vi "Omron Serial FINS-Command Frame.vi"(8 "error in":errorcluster, 10 "FINS Command Frame":T3 {"Response Wait Time" items=["0 ms", "10 ms", "20 ms", "30 ms", "40 ms", "50 ms", "60 ms", "70 ms", "80 ms", "90 ms", "100 ms", "110 ms", "120 ms", "130 ms", "140 ms", "150 ms"]}, 11 "Buffer Data In":T1={"VISA Resource Name"="", "Wait For Read(ms)"=50, "Command Code"=enum."Memory area read", "Command String"="", "Read Bytes"=0, "Response String"=""}) -> (0 "error out":errorcluster, 3 "Buffer Data Out":T1={"VISA Resource Name"="", "Wait For Read(ms)"=50, "Command Code"=enum."Memory area read", "Command String"="", "Read Bytes"=0, "Response String"=""})   [LabVIEW 2016]
uses:
  Data Def/Omron Serial FINS-FINS Command Frame.ctl
  Data Def/Omron Serial FINS-Command Code.ctl
  Data Def/Omron Serial FINS-Buffer Data.ctl
  Data Def/Omron Serial FINS-Memory Area Read Data.ctl
  Data Def/Omron Serial FINS-Memory Area Write Data.ctl
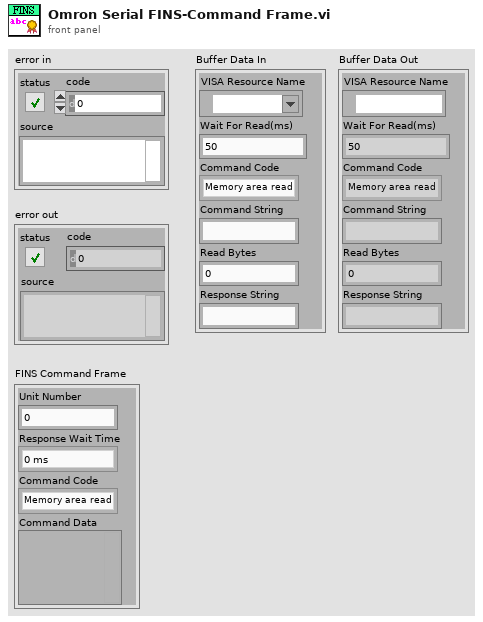
[diagram p1: front panel]
types:
  T1 = typedef "Omron Serial FINS-Buffer Data.ctl" = cluster{"VISA Resource Name":refnum<visa-resource-name>, "Wait For Read(ms)":u32, "Command Code":T2, "Command String":string, "Read Bytes":u32, "Response String":string}
  T2 = typedef "Omron Serial FINS-Command Code.ctl" = enum16{"Memory area read", "Memory area write"}
  T3 = typedef "Omron Serial FINS-FINS Command Frame.ctl" = cluster{"Unit Number":u8, "Response Wait Time":u8, "Command Code":T2, "Command Data":variant}
  T4 = typedef "Omron Serial FINS-Memory Area Read Data.ctl" = cluster{"I/O Memory Address":i32, "Beginning Address":u32, "No. Of Items":u32}
  T5 = typedef "Omron Serial FINS-Memory Area Write Data.ctl" = cluster{"I/O Memory Address":i32, "Beginning Address":u32, "No. Of Items":u32, "Data":i16[]}
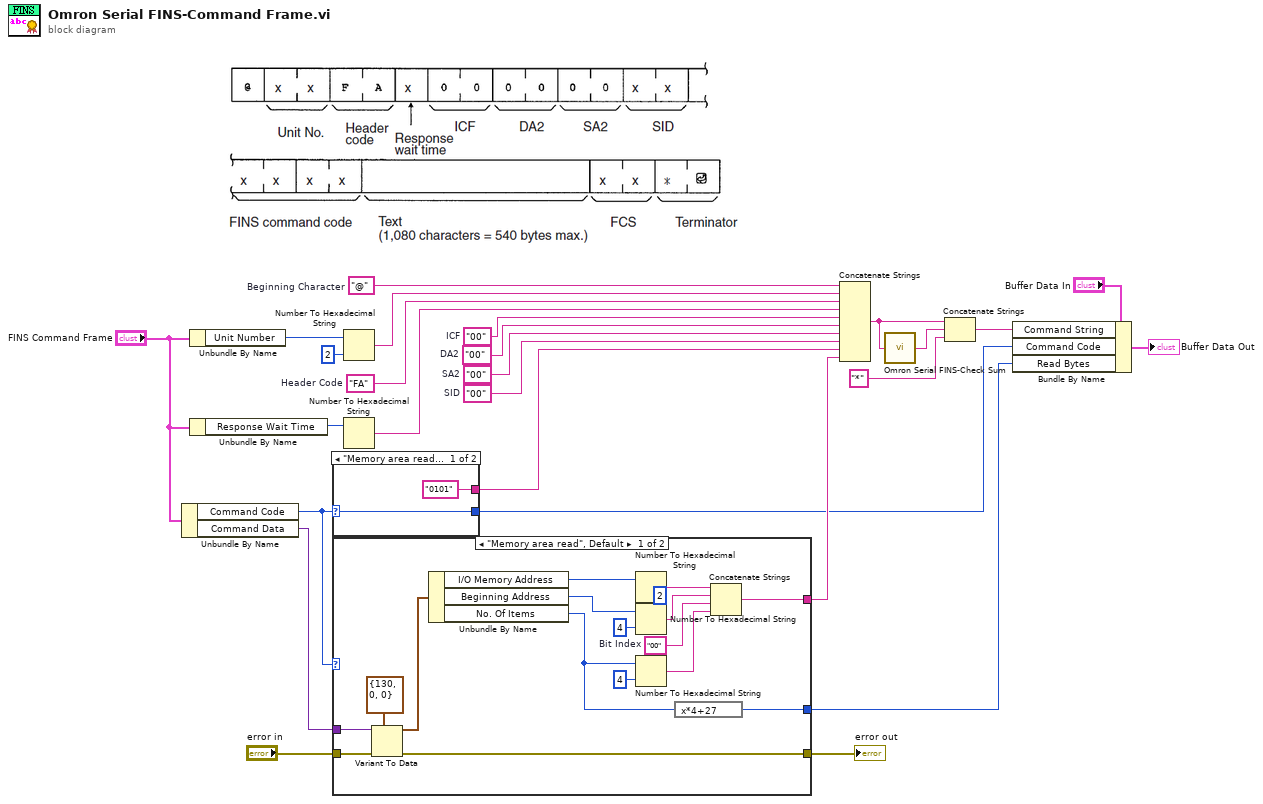
[diagram p0: block diagram]
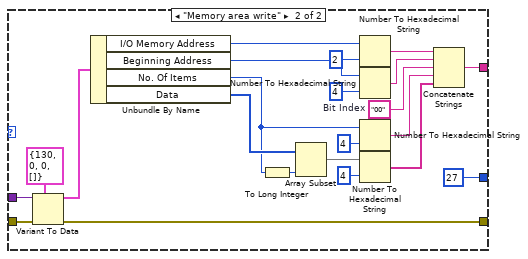
[diagram p2: hidden frame]
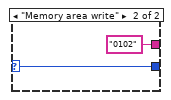
[diagram p3: hidden frame]
diagram:
  w17 = "00"  # SID
  w18 = "00"  # SA2
  w19 = "00"  # DA2
  w3 = "00"  # ICF
  w25 = "FA"  # Header Code
  w26 = "@"  # Beginning Character
  n1 = Unbundle By Name("FINS Command Frame") -> ("Command Code"=w15:T2, "Command Data"=w14:variant)
  n2 = Unbundle By Name("FINS Command Frame") -> ("Unit Number"=w24:u8)
  n3 = Unbundle By Name("FINS Command Frame") -> ("Response Wait Time"=w21:u8)
  n4 = case shown="\"Memory area read\", Default" w15 {
    selector: w15 -> [w27 w29]
    tunnel: ["0101" ("Command code") "0102" ("Command code")] -> w16
    tunnel: [w27 w29] -> w2
    frame "Memory area read", Default {
    }
    frame "Memory area write" {
    }
  }
  n5 = case shown="\"Memory area read\", Default" w15 {
    tunnel: w14 -> [w46 w68]
    tunnel: "error in" -> [w47 w69]
    tunnel: [w41 w64] -> w12
    tunnel: [w33 w58] -> w11
    tunnel: [w31 u32 27 ("No. Of Items")] -> w1
    frame "Memory area read", Default {
      w36 = "00"  # Bit Index
      n6 = Variant To Data(error in=w47, type=T4 {"I/O Memory Address"=130, "Beginning Address"=0, "No. Of Items"=0} ("Memory Area Read Data"), Variant=w46) -> (data=w44:T4, error out=w41:errorcluster)
      n7 = Unbundle By Name(w44) -> ("I/O Memory Address"=w43:i32, "Beginning Address"=w39:u32, "No. Of Items"=w32:u32)
      n8 = Number To Hexadecimal String(1:i16 2 ("width (-)"), 2:w43) -> (0:w38:string)
      n9 = Number To Hexadecimal String(1:i16 4 ("width (-)"), 2:w39) -> (0:w37:string)
      n10 = Number To Hexadecimal String(1:i16 4 ("width (-)"), 2:w32) -> (0:w34:string)
      n11 = expression code="x*4+27"(w32) -> (w31:u32)
      n12 = Concatenate Strings(w38, w37, w36, w34) -> (w33:string)
    }
    frame "Memory area write" {
      w61 = "00"  # Bit Index
      n13 = Variant To Data(error in=w69, type=T5 {"I/O Memory Address"=130, "Beginning Address"=0, "No. Of Items"=0, "Data"=[]} ("Memory Area Write Data"), Variant=w68) -> (data=w67:T5, error out=w64:errorcluster)
      n14 = Unbundle By Name(w67) -> ("I/O Memory Address"=w66:i32, "Beginning Address"=w53:u32, "No. Of Items"=w49:u32, "Data"=w52:i16[])
      n15 = To Long Integer(number=w49) -> (32bit integer=w50:i32)
      n16 = Array Subset(array=w52, length=w50) -> (w51:i16[])  [unwired: 1 in]
      n17 = Number To Hexadecimal String(1:i16 2 ("width (-)"), 2:w66) -> (0:w63:string)
      n18 = Number To Hexadecimal String(1:i16 4 ("width (-)"), 2:w53) -> (0:w62:string)
      n19 = Number To Hexadecimal String(1:i16 4 ("width (-)"), 2:w49) -> (0:w59:string)
      n20 = Number To Hexadecimal String(1:i16 4 ("width (-)"), 2:w51) -> (0:w55:string[])
      n21 = Concatenate Strings(w63, w62, w61, w59, w55) -> (w58:string)
    }
  }
  "error out" <- w12
  n22 = Number To Hexadecimal String(1:i16 2 ("width (-)"), 2:w24) -> (0:w22:string)
  n23 = Number To Hexadecimal String(2:w21) -> (0:w20:string)  [unwired: 1 in]
  n24 = Concatenate Strings(w26, w22, w25, w20, w3, w19, w18, w17, w16, w11) -> (w9:string)
  n25 = call "Omron Serial FINS-Check Sum.vi"("Check String"=w9) -> ("FCS"=w10:string)
  n26 = Concatenate Strings(w9, w10, "*" ("string")) -> (w6:string)
  n27 = Bundle By Name(cluster="Buffer Data In", "Command String"=w6, "Command Code"=w2, "Read Bytes"=w1) -> (→"Buffer Data Out":T1)
